vi "Build Message Configuration.vi"(7 "Virtual Memory Unit in":refnum<class "Virtual Memory Unit.lvclass">, 8 "error in (no error)":errorcluster, 10 "Starting Address":u16 format="%04x", 11 "Message in":refnum<class "Message.lvclass">) -> (0 "error out":errorcluster, 2 "Next Available Address":u16 format="%04x", 3 "Message out":refnum<class "Message.lvclass">, 5 "Virtual Memory Unit out":refnum<class "Virtual Memory Unit.lvclass">)   [LabVIEW 2020, in "BCI-1553 API.lvlib" / "Message.lvclass"]
doc: "Builds the message control and status blocks. Regardless of message type, this block should always be 16 registers long."
uses:
  Message.lvclass
  Dependencies/Virtual Memory Unit/Virtual Memory Unit.lvclass
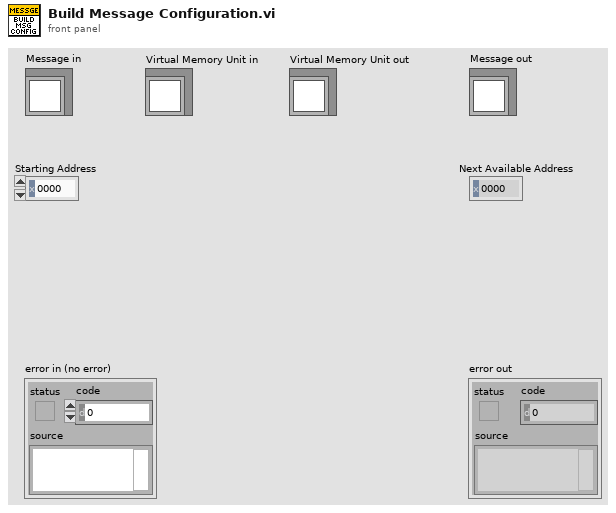
[diagram p1: front panel]
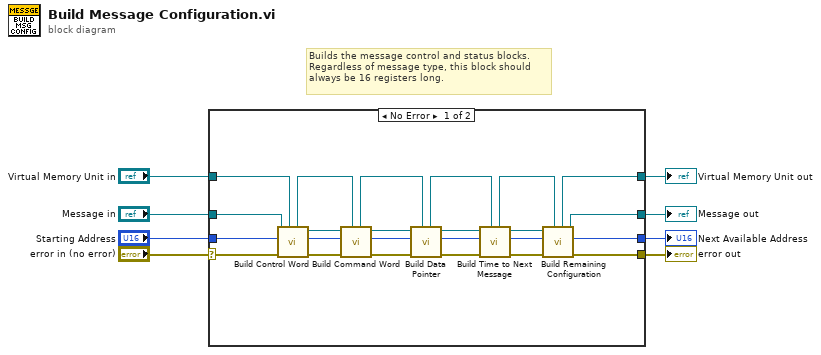
[diagram p0: block diagram]
diagram:
  # "Builds the message control and status blocks.\nRegardless of message type, this block should\nalways be 16 registers long."
  n1 = case shown="No Error" "error in (no error)" {
    selector: "error in (no error)" -> [w32 w36]
    tunnel: [w9 w36] -> w7
    tunnel: [w14 w35] -> w5
    tunnel: "Message in" -> [w31 w35]
    tunnel: "Starting Address" -> [w29 w34]
    tunnel: "Virtual Memory Unit in" -> [w30 w33]
    tunnel: [w12 w34] -> w2
    tunnel: [w16 w33] -> w1
    frame No Error {
      n2 = call-dynamic "Build Control Word.vi"("Virtual Memory Unit in"=w30, "error in (no error)"=w32, "Starting Address"=w29, "Message in"=w31) -> ("error out"=w26:errorcluster, "Next Available Address"=w25:u16, "Message out"=w27:refnum<class "Message.lvclass">, "Virtual Memory Unit out"=w28:refnum<class "Virtual Memory Unit.lvclass">)  [unwired: 4 in]
      n3 = call-dynamic "Build Command Word.vi"("Virtual Memory Unit in"=w28, "error in (no error)"=w26, "Starting Address"=w25, "Message in"=w27) -> ("error out"=w10:errorcluster, "Next Available Address"=w13:u16, "Message out"=w15:refnum<class "Message.lvclass">, "Virtual Memory Unit out"=w24:refnum<class "Virtual Memory Unit.lvclass">)  [unwired: 4 in]
      n4 = call-dynamic "Build Data Pointer.vi"("Virtual Memory Unit in"=w24, "error in (no error)"=w10, "Starting Address"=w13, "Message in"=w15) -> ("error out"=w21:errorcluster, "Next Available Address"=w22:u16, "Message out"=w23:refnum<class "Message.lvclass">, "Virtual Memory Unit out"=w20:refnum<class "Virtual Memory Unit.lvclass">)  [unwired: 4 in]
      n5 = call-dynamic "Build Time to Next Message.vi"("Virtual Memory Unit in"=w20, "error in (no error)"=w21, "Starting Address"=w22, "Message in"=w23) -> ("error out"=w11:errorcluster, "Next Available Address"=w18:u16, "Message out"=w19:refnum<class "Message.lvclass">, "Virtual Memory Unit out"=w17:refnum<class "Virtual Memory Unit.lvclass">)  [unwired: 4 in]
      n6 = call-dynamic "Build Remaining Configuration.vi"("Virtual Memory Unit in"=w17, "error in (no error)"=w11, "Starting Address"=w18, "Message in"=w19) -> ("error out"=w9:errorcluster, "Next Available Address"=w12:u16, "Message out"=w14:refnum<class "Message.lvclass">, "Virtual Memory Unit out"=w16:refnum<class "Virtual Memory Unit.lvclass">)  [unwired: 4 in]
    }
    frame Error {
    }
  }
  "error out" <- w7
  "Message out" <- w5
  "Virtual Memory Unit out" <- w1
  "Next Available Address" <- w2
